vi "Valid Answers--constant.vi"() -> (3 "Valid Answers":set{string}(c389))   [LabVIEW 2020, in "Wordle Engine.lvlib"]
uses:
  Wordle Engine.lvlib
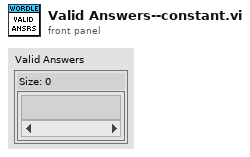
[diagram p1: front panel]
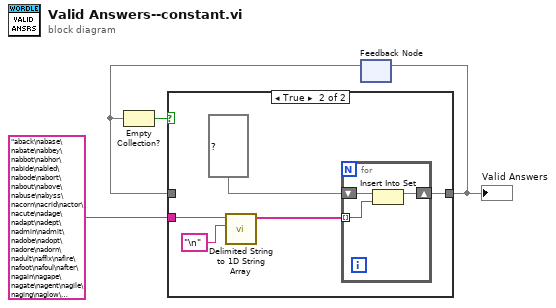
[diagram p0: block diagram]
diagram:
  n1 = feedback #1() -> (w2:set{string})  [unwired: 1 in]
  n2 = Empty Collection?(1:w2) -> (0:w4:bool)
  n3 = case shown="True" w4 {
    tunnel: "aback\nabase\nabate\nabbey\nabbot\nabhor\nabide\nabled\nabode\nabort\nabout\nabove\nabuse\nabyss\nacorn\nacrid\nactor\nacute\nadage\nadapt\nadept\nadmin\nadmit\nadobe\nadopt\nadore\nadorn\nadult\naffix\nafire\nafoot\nafoul\nafter\nagain\nagape\nagate\nagent\nagile\naging\naglow\nagony\nagora\nagree\nahead\naider\naisle\nalarm\nalbum\nalert\nalgae\nalibi\nalien\nalign\nalike\nalive\nallay\nalley\nallot\nallow\nalloy\naloft\nalone\nalong\naloof\naloud\nalpha\naltar\nalter\namass\namaze\namber\namble\namend\namiss\namity\namong\nample\namply\namuse\nangel\nanger\nangle\nangry\nangst\nanime\nankle\nannex\nannoy\nannul\nanode\nantic\nanvil\naorta\napart\naphid\naping\napnea\napple\napply\napron\n..." -> [_ w10]
    tunnel: [w5 w7] -> w1
    tunnel: w2 -> [w5 _]
    frame False {
    }
    frame True {
      n4 = call <vilib>:"Delimited String to 1D String Array.vi"("delimiter"="\n", "delimited string"=w10) -> ("string array"=w9:string[])  [unwired: 9 in]
      n5 = for {
        tunnel: w9 -> [w11] mode=indexing
        shift-right: [w13] -> w7
        shift-left: set{string} {} ("Valid Guesses") -> [w12]
        n6 = Insert Into Set(10:w11, 11:w12) -> (3:w13:set{string})  [unwired: 1 out]
      }
    }
  }
  "Valid Answers" <- w1
  n7 = feedback-in #1(w1) -> ()
